vi "db_transactions_insert.vi"(0 "UDL PATH IN":path, 1 "TABLE NAME":string, 2 "FIELDS (if any)":string[](array[string]), 4 "VALUES":string[](array[string]), 5 "ERROR IN":errorcluster) -> (14 "UDL PATH OUT":path, 19 "ERROR OUT":errorcluster)   [LabVIEW 2018, in "db_lib R3.lvlib"]
uses:
  db_lib R3.lvlib
  <vilib>/addons/database/Connection.llb/DB Tools Open Connec (Path).vi
  <vilib>/addons/database/Connection.llb/Conn Execute.vi
  <vilib>/addons/database/Recordset.llb/Rec Destroy - Connection.vi
  <vilib>/addons/database/NI_Database_API.lvlib
panel:
  # "INSERT INTO [table_name](fields) VALUES [data];"
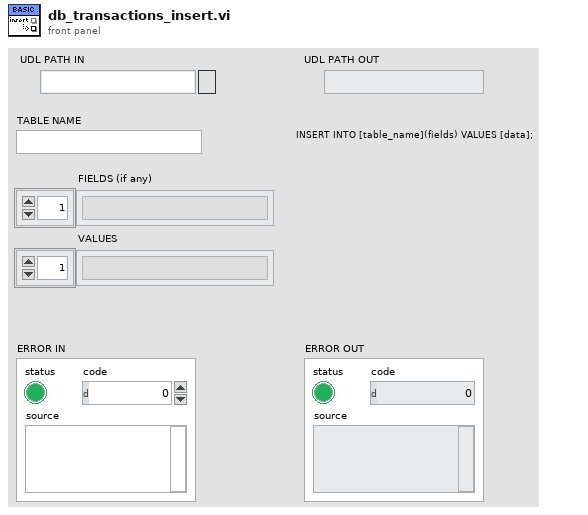
[diagram p1: front panel]
types:
  T1 = typedef "NI_Database_API.lvlib/Conn ObjectReference.ctl" = refnum<k1>
  T2 = typedef "NI_Database_API.lvlib/Rec ObjectReference.ctl" = refnum<k1>
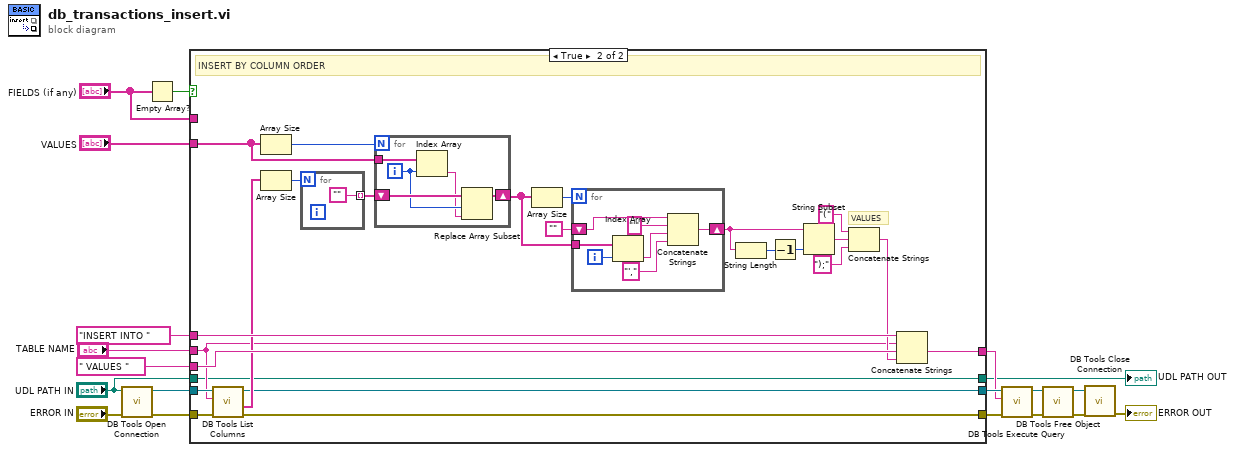
[diagram p0: block diagram]
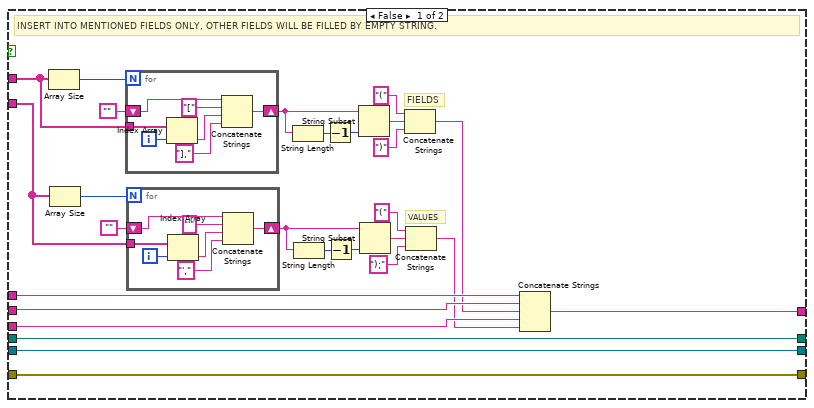
[diagram p2: hidden frame]
diagram:
  n1 = call-poly <vilib>:"DB Tools Open Connection.vi"("error in (no error)"="ERROR IN", "connection information"="UDL PATH IN") -> ("error out"=w15:errorcluster, "connection reference"=w14:T1)  [unwired: 6 in]
  n2 = Empty Array?(array="FIELDS (if any)") -> (empty?=w5:bool)
  n3 = case shown="True" w5 {
    tunnel: "INSERT INTO " -> [w28 w84]
    tunnel: " VALUES " -> [w25 w83]
    tunnel: w15 -> [w21 w82]
    tunnel: w14 -> [w22 w81]
    tunnel: "VALUES" -> [w31 w80]
    tunnel: [w22 w77] -> w8
    tunnel: [w21 w76] -> w7
    tunnel: [w23 w64] -> w6
    tunnel: "TABLE NAME" -> [w27 w63]
    tunnel: "FIELDS (if any)" -> [w46 _]
    tunnel: "UDL PATH IN" -> [w20 w61]
    tunnel: [w20 w61] -> w1
    frame False {
      # "VALUES"
      # "FIELDS"
      # "INSERT INTO MENTIONED FIELDS ONLY, OTHER FIELDS WILL BE FILLED BY EMPTY STRING."
      n4 = Array Size(array=w46) -> (size(s)=w29:i32)
      n5 = Array Size(array=w31) -> (size(s)=w30:i32)
      n6 = for {
        N: w29 -> [_]
        tunnel: w46 -> [w60]
        shift-right: [w55] -> w44
        shift-left: "" -> [w54]
        i -> [w59]
        n7 = Index Array(array=w60, index=w59) -> (element=w57:string)
        n8 = Concatenate Strings(w54, "[" ("string"), w57, "]," ("string")) -> (w55:string)
      }
      n9 = for {
        N: w30 -> [_]
        tunnel: w31 -> [w53]
        shift-right: [w48] -> w37
        shift-left: "" -> [w47]
        i -> [w52]
        n10 = Index Array(array=w53, index=w52) -> (element=w50:string)
        n11 = Concatenate Strings(w47, "'" ("string"), w50, "'," ("string")) -> (w48:string)
      }
      n12 = String Length(string=w44) -> (length=w43:i32)
      n13 = String Length(string=w37) -> (length=w36:i32)
      n14 = Decrement(x=w43) -> (x-1=w42:i32)
      n15 = Decrement(x=w36) -> (x-1=w35:i32)
      n16 = String Subset(string=w44, length (rest)=w42) -> (substring=w41:string)  [unwired: 1 in]
      n17 = String Subset(string=w37, length (rest)=w35) -> (substring=w34:string)  [unwired: 1 in]
      n18 = Concatenate Strings("(" ("string"), w41, ")" ("string")) -> (w26:string)
      n19 = Concatenate Strings("(" ("string"), w34, ");" ("string")) -> (w24:string)
      n20 = Concatenate Strings(w28, w27, w26, w25, w24) -> (w23:string)
    }
    frame True {
      # "VALUES"
      # "INSERT BY COLUMN ORDER"
      n21 = call <vilib>:"DB Tools List Columns.vi"("error in (no error)"=w82, "table"=w63, "connection reference"=w81) -> ("error out"=w76:errorcluster, "columns"=w79:string[], "connection reference out"=w77:T1)  [unwired: 1 in, 1 out]
      n22 = Array Size(array=w80) -> (size(s)=w75:i32)
      n23 = Array Size(array=w79) -> (size(s)=w62:i32)
      n24 = for {
        N: w62 -> [_]
        tunnel: [""] -> w78 mode=indexing
      }
      n25 = for {
        N: w75 -> [_]
        tunnel: w80 -> [w96]
        shift-right: [w92] -> w72
        shift-left: w78 -> [w95]
        i -> [w94]
        n26 = Index Array(array=w96, index=w94) -> (element=w93:string)
        n27 = Replace Array Subset(array=w95, new element=w93, index=w94) -> (w92:string[])
      }
      n28 = Array Size(array=w72) -> (size(s)=w74:i32)
      n29 = for {
        N: w74 -> [_]
        tunnel: w72 -> [w91]
        shift-right: [w86] -> w69
        shift-left: "" -> [w85]
        i -> [w90]
        n30 = Index Array(array=w91, index=w90) -> (element=w88:string)
        n31 = Concatenate Strings(w85, "'" ("string"), w88, "'," ("string")) -> (w86:string)
      }
      n32 = String Length(string=w69) -> (length=w71:i32)
      n33 = Decrement(x=w71) -> (x-1=w70:i32)
      n34 = String Subset(string=w69, length (rest)=w70) -> (substring=w68:string)  [unwired: 1 in]
      n35 = Concatenate Strings("(" ("string"), w68, ");" ("string")) -> (w65:string)
      n36 = Concatenate Strings(w84, w63, w83, w65) -> (w64:string)
    }
  }
  "UDL PATH OUT" <- w1
  n37 = call-poly <vilib>:"DB Tools Execute Query.vi"("error in (no error)"=w7, "SQL query"=w6, "connection reference"=w8) -> ("error out"=w10:errorcluster, "recordset reference"=w9:T2)  [unwired: 5 in]
  n38 = call-poly <vilib>:"DB Tools Free Object.vi"("error in (no error)"=w10, "recordset reference"=w9) -> ("error out"=w13:errorcluster, "connection reference"=w12:T1)  [unwired: 8 in]
  n39 = call <vilib>:"DB Tools Close Connection.vi"("error in (no error)"=w13, "connection reference"=w12) -> ("error out"=→"ERROR OUT":errorcluster)  [unwired: 5 in]
